vi "NI 9215 TSN Sync(FPGA).vi"() -> ()   [LabVIEW 2018]
uses:
  <vilib>/Platform/TimedLoop/XDataNode/timing_clust.ctl
  <vilib>/Platform/TimedLoop/XDataNode/nitl_modes.ctl
  <vilib>/Platform/TimedLoop/XDataNode/wakeup.ctl
  <vilib>/rvi/Emulation/niFpgaGetClockAttributes.vi
  <vilib>/rvi/Emulation/niFpgaSctlEmulationGetInTimedLoop.vi
  <vilib>/rvi/Emulation/niFpgaEmulationReportErrorSimple.vi
  <vilib>/rvi/Emulation/niFpgaCriticalErrorInLSC.vi
  <vilib>/rvi/eio/common/nirviEmuTemplateMethod_errors.vi
  <vilib>/rvi/interface/RandomDataEmulation/niFpgaRandomDataHandleErrors.vi
  <vilib>/Platform/TimedLoop/XDataNode/XDataNode.xnode
  <vilib>/eio/EIONode/EIONode.xnode
  <vilib>/rvi/DataTransferAndStorage/Container/XNode/niFpgaContainer.xnode
  <vilib>/rvi/interface/RandomDataEmulation/nirviRandomDataFpgaReadWriteTemplate.vi
  <vilib>/Platform/TimedLoop/XDataNode/XDNodeRunTimeDep.lvlib
panel:
  out "FPGA Error Out":errorcluster
  out "Data FIFO Full":bool
  out "Loop Iterations":i32
  out "Curr Time":u64
  in  "Set Start Time":bool
  in  "Sample Period (ns)":u32=20
  in  "Acquisition Start Time":u64=18446744073709551615
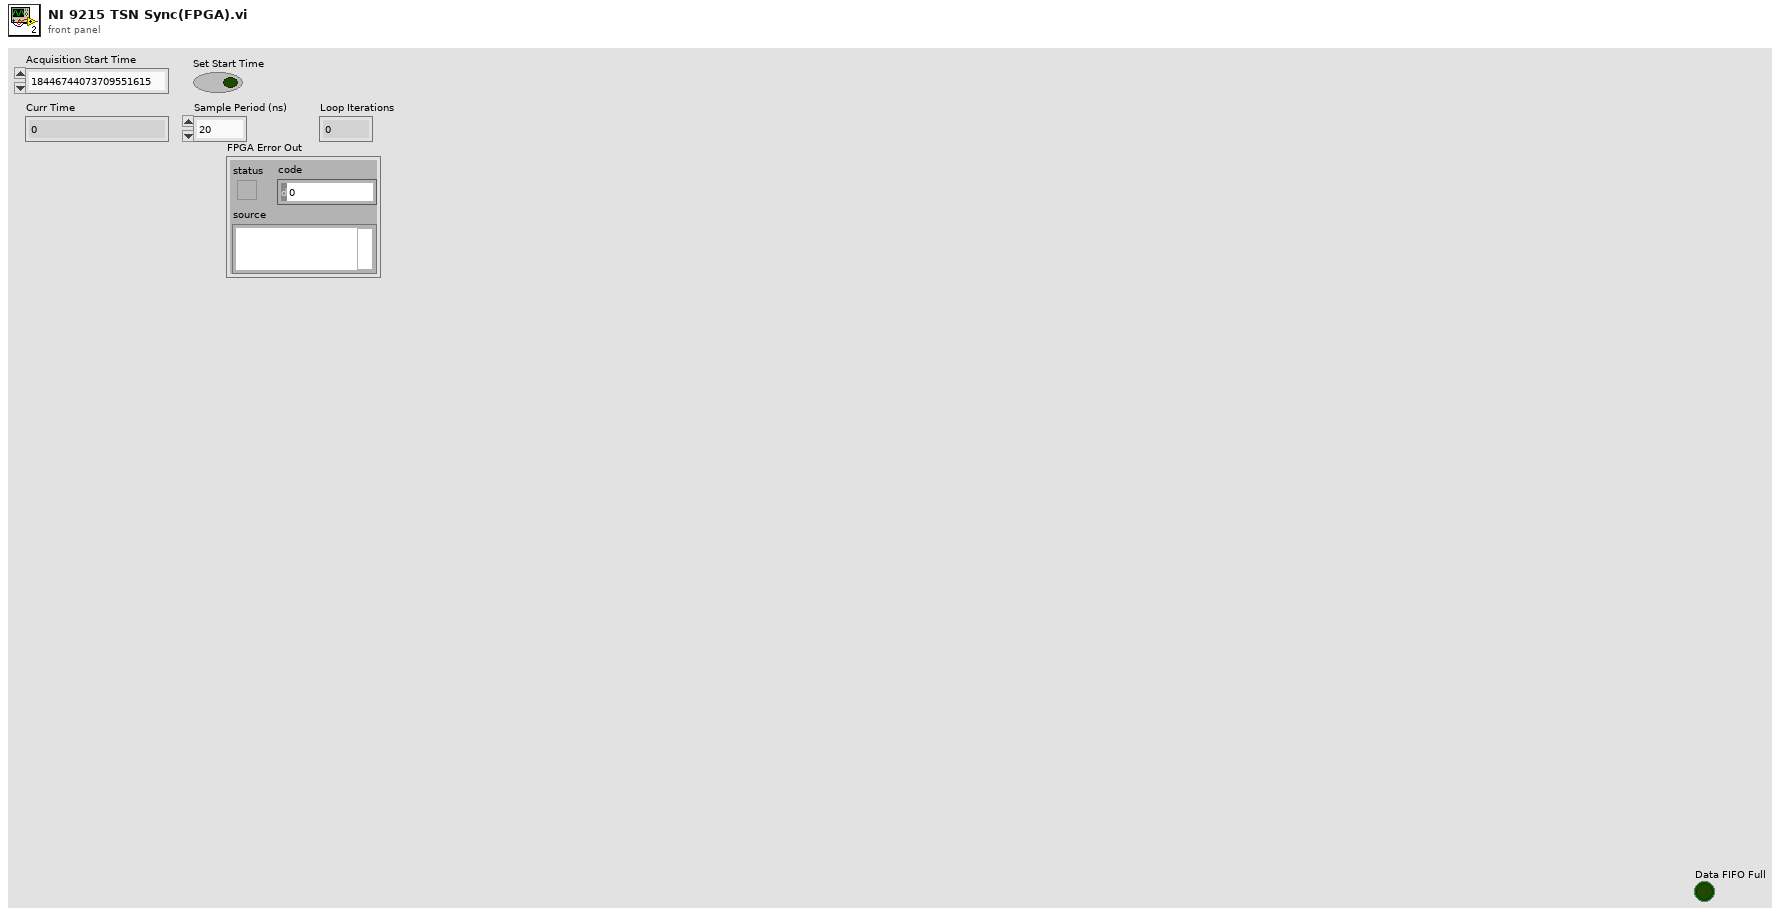
[diagram p1: front panel]
types:
  T1 = typedef "XDNodeRunTimeDep.lvlib/timing_clust.ctl" = cluster{"Expected End [f-1]":u64, "Actual End [f-1]":u64, "Finished Late? [f-1]":bool, "Expected End [i-1]":u64, "Actual End [i-1]":u64, "Finished Late? [i-1]":bool, "Expected Start [i]":u64, "Actual Start [i]":u64, "Expected Start [f]":u64, "Actual Start [f]":u64, "Source Name":string, "Structure Name":string, "Period":i64, "Deadline":i64, "Offset":i64, "Start":i64, "Priority":i32, "Timeout":i32, "Mode":T2, "Wakeup Reason":T3, "Error":errorcluster, "Source Type":string, "Secondary Source Type":string, "Global End Time":u64, "Global Start Time":u64, "Frame Duration":u64, "Iteration Duration":u64, "Assigned CPU":i32, "I/O Scan Engine Mode":u32}
  T2 = typedef "XDNodeRunTimeDep.lvlib/nitl_modes.ctl" = enum32{"No Change", "Process missed periods, maintain original phase", "Discard missed periods, maintain original phase", "Process missed periods, ignore original phase", "Discard missed periods, ignore original phase"}
  T3 = typedef "XDNodeRunTimeDep.lvlib/wakeup.ctl" = enum32{"Normal", "Aborted", "Asynchronous wakeup", "Timing source error", "Timed loop error", "Timeout"}
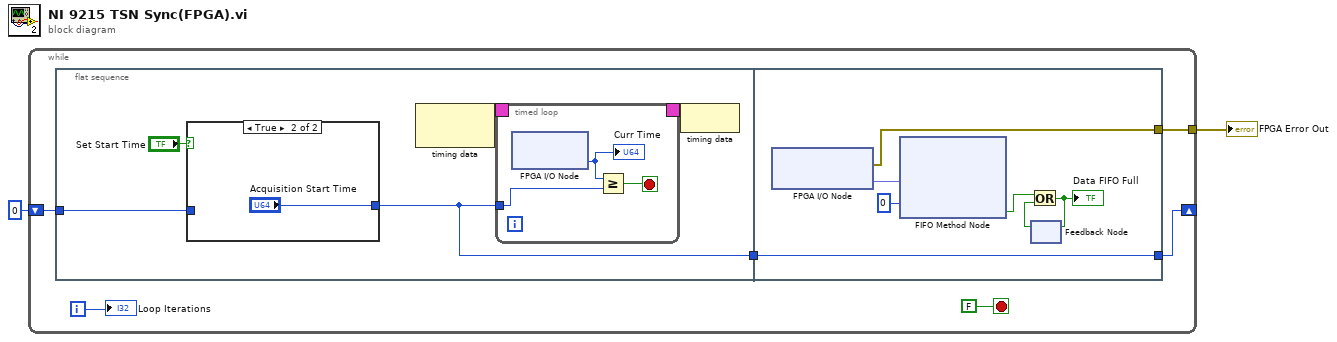
[diagram p0: block diagram]
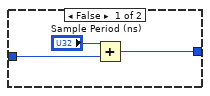
[diagram p2: hidden frame]
diagram:
  n1 = while {
    shift-right: [w4] -> _
    shift-left: u64 0 ("Update Period (ns)") -> [w6]
    tunnel: [w3] -> w1
    i -> [w7]
    stop <- FALSE stop-if-true
    n2 = flat-sequence {
      tunnel: w6 -> [w10]
      tunnel: [w9] -> w5
      tunnel: w5 -> [w30]
      tunnel: [w30] -> w4
      tunnel: [w25] -> w3
      frame #0 {
        n3 = case shown="True" "Set Start Time" {
          tunnel: [w14 "Acquisition Start Time"] -> w9
          tunnel: w10 -> [w15 _]
          frame False {
            n4 = Add(x="Sample Period (ns)", y=w15) -> (x+y=w14:u64)
          }
          frame True {
          }
        }
        n5 = node-c288() -> (w13:T1)  [unwired: 1 in]
        n6 = timed-loop {
          timing: w13 -> [_]
          timing-out: [_] -> w12
          tunnel: w9 -> [w18]
          stop <- w19 stop-if-true
          n7 = xnode "FPGA I/O Node"() -> ("Time"=w20:u64)  [unwired: 1 in, 1 out]
          "Curr Time" <- w20
          n8 = Greater Or Equal?(x=w20, y=w18) -> (x >= y?=w19:bool)
        }
        n9 = node-c288(w12) -> ()
      }
      frame #1 {
        n10 = xnode "FPGA I/O Node"() -> ("error out"=w25:errorcluster, "Mod1/AI0"=w31:fxp<+/-,20,5>)  [unwired: 2 in, 1 out]
        n11 = xnode ("FIFO Method Node")("Element"=w31, "Timeout"=0) -> ("Timed Out?"=w27:bool)  [unwired: 1 in, 1 out]
        n12 = feedback #1() -> (w26:bool)  [unwired: 1 out]
        n13 = Or(x=w27, y=w26) -> (x .or. y?=w28:bool)
        "Data FIFO Full" <- w28
        n14 = feedback-in #1(w28) -> ()
      }
    }
    "Loop Iterations" <- w7
  }
  "FPGA Error Out" <- w1
